vi "GetTurretAngle.vi"(2 "Robot Heading (deg)":dbl) -> (0 "Turret Heading (deg)":dbl, 1 "Turret Angle (deg)":dbl)   [LabVIEW 2020]
doc: "Gets the current turret angle relative to the robot and the turret heading in field coordinates."
uses:
  sensordata.vi
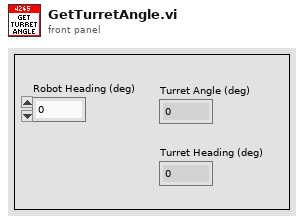
[diagram p1: front panel]
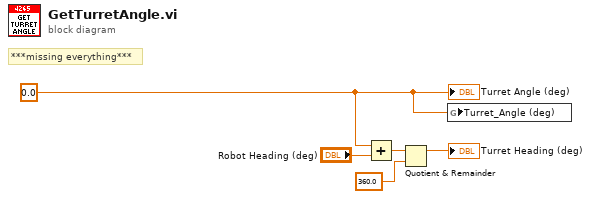
[diagram p0: block diagram]
diagram:
  w1 = 0.0 ("Turret Angle (deg)")
  # "***missing everything***"
  n1 = Add(x=w1, y="Robot Heading (deg)") -> (x+y=w4:dbl)
  n2 = Quotient & Remainder(x=w4, y=360.0) -> (x-y*floor(x/y)=→"Turret Heading (deg)":dbl)  [unwired: 1 out]
  n3 = global write "sensordata.vi" "Turret_Angle (deg)"(w1) -> ()
  "Turret Angle (deg)" <- w1
